vi "读取数值.vi"(8 "error in (no error)":errorcluster, 10 "Slave ID":u8=1, 11 "MB session in":refnum<class "MB_Master.lvclass">) -> (0 "error out":errorcluster, 2 "读取值":T1, 3 "MB session out":refnum<class "MB_Master.lvclass">)   [LabVIEW 2016, in "流量计集成.lvlib" / "博意达流量计.lvlib"]
uses:
  <vilib>/Plasmionique/MB Master/MB_Master/MB_Master.lvclass
  <vilib>/Plasmionique/MB Master/MB Master.lvlib
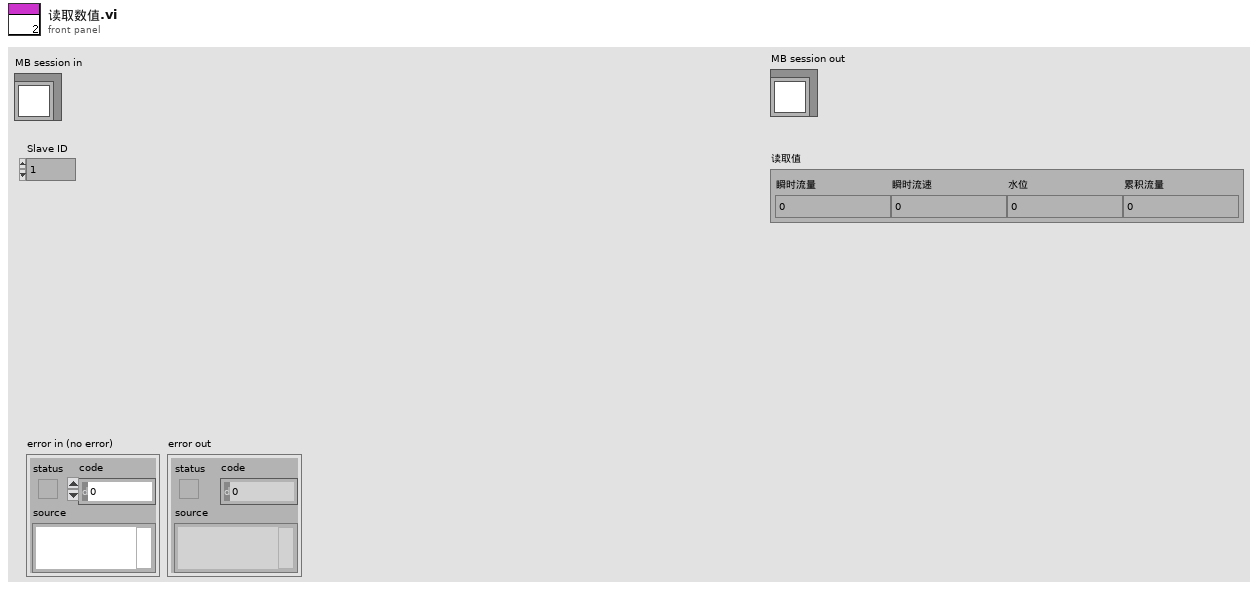
[diagram p1: front panel]
types:
  T1 = typedef "流量计集成.lvlib/博意达流量计.lvlib/读取值.ctl" = cluster{"瞬时流量":sgl, "瞬时流速":sgl, "水位":sgl, "累积流量":sgl}
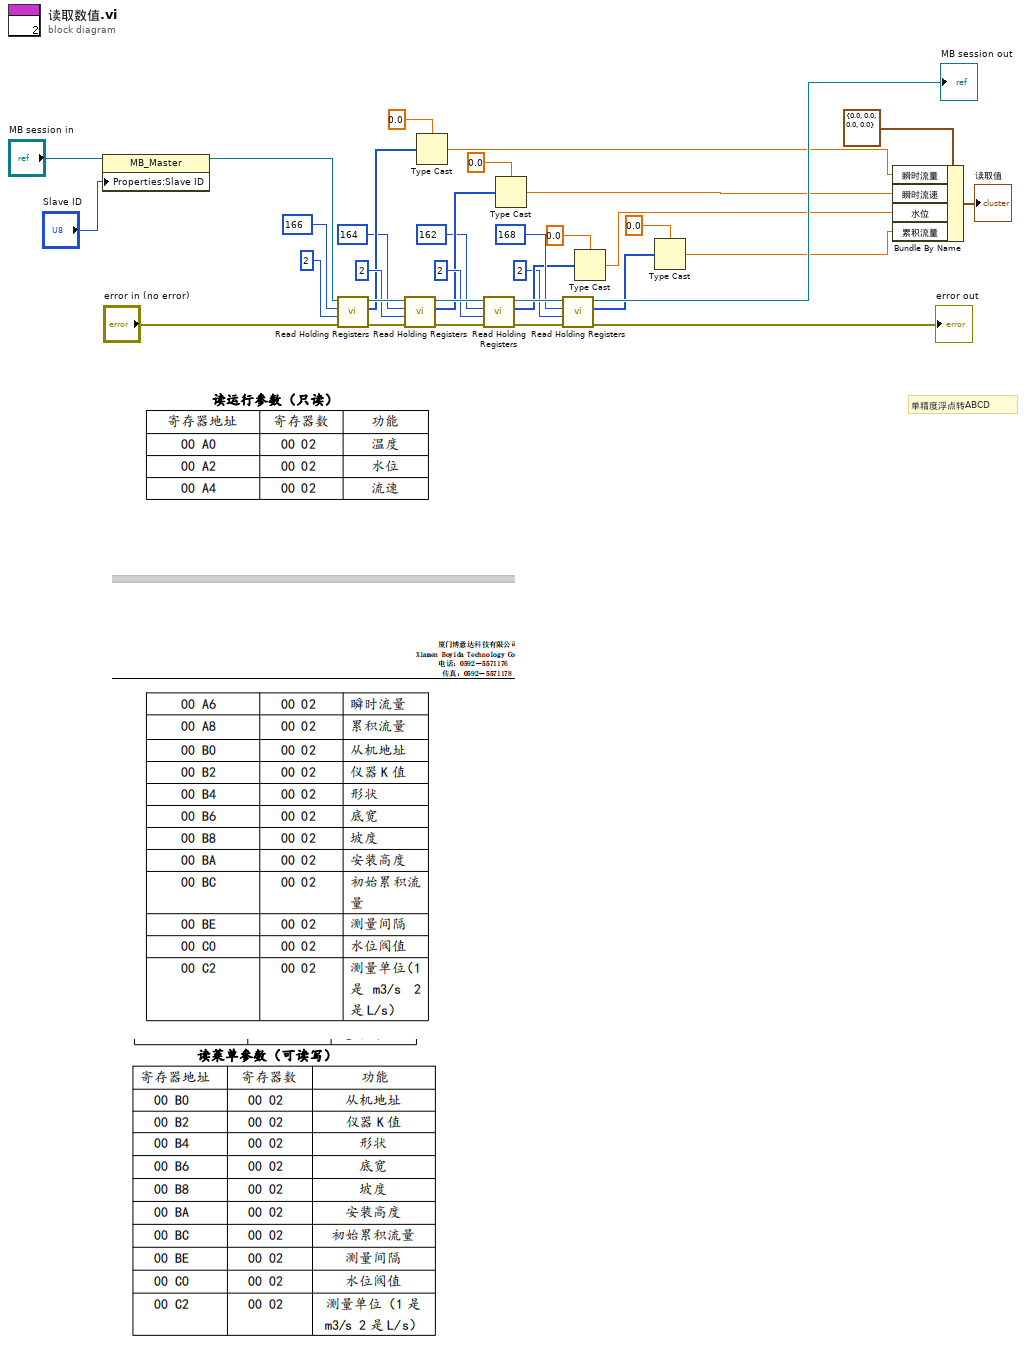
[diagram p0: block diagram]
diagram:
  # "单精度浮点转ABCD"
  n1 = property class="MB_Master"(reference="MB session in", "Properties:Slave ID"="Slave ID") -> (reference out=w20:refnum<class "MB_Master.lvclass">)  [unwired: 1 in, 1 out]
  n2 = call <vilib>:"Read Holding Registers.vi"("error in (no error)"="error in (no error)", "quantity"=u16 2, "starting address"=u16 166, "MB session in"=w20) -> ("error out"=w32:errorcluster, "Registers"=w24:u16[], "MB session out"=w33:refnum<class "MB_Master.lvclass">)  [unwired: 5 in]
  n3 = call <vilib>:"Read Holding Registers.vi"("error in (no error)"=w32, "quantity"=u16 2, "starting address"=u16 164, "MB session in"=w33) -> ("error out"=w28:errorcluster, "Registers"=w23:u16[], "MB session out"=w30:refnum<class "MB_Master.lvclass">)  [unwired: 5 in]
  n4 = Type Cast(type=sgl 0.0 ("x/y"), x=w24) -> (*(type *) &x=w1:sgl)
  n5 = call <vilib>:"Read Holding Registers.vi"("error in (no error)"=w28, "quantity"=u16 2, "starting address"=u16 162, "MB session in"=w30) -> ("error out"=w26:errorcluster, "Registers"=w22:u16[], "MB session out"=w27:refnum<class "MB_Master.lvclass">)  [unwired: 5 in]
  n6 = Type Cast(type=sgl 0.0 ("x/y"), x=w23) -> (*(type *) &x=w3:sgl)
  n7 = call <vilib>:"Read Holding Registers.vi"("error in (no error)"=w26, "quantity"=u16 2, "starting address"=u16 168, "MB session in"=w27) -> ("error out"=→"error out":errorcluster, "Registers"=w8:u16[], "MB session out"=→"MB session out":refnum<class "MB_Master.lvclass">)  [unwired: 5 in]
  n8 = Type Cast(type=sgl 0.0 ("x/y"), x=w22) -> (*(type *) &x=w5:sgl)
  n9 = Type Cast(type=sgl 0.0 ("x/y"), x=w8) -> (*(type *) &x=w7:sgl)
  n10 = Bundle By Name(cluster=T1 {"瞬时流量"=0.0, "瞬时流速"=0.0, "水位"=0.0, "累积流量"=0.0} ("读取值"), "瞬时流量"=w1, "瞬时流速"=w3, "水位"=w5, "累积流量"=w7) -> (→"读取值":T1)
